vi "InitIntensityGraph.vi"(8 "error in (no error)":errorcluster, 11 "IntensityGraph in":refnum<vi>) -> (0 "error out":errorcluster, 3 "IntensityGraph out":refnum<vi>)   [LabVIEW 2023]
doc: "This VI setups the intensity map and fills it with generated test data for the purpose of this demo."
panel:
  out "appended array":dbl[][](array[numeric])
  in  "Number Y":i32
  in  "StartY":dbl=-0.5
  in  "NumberX":i32
  in  "StartX":dbl=-0.5
  in  "r":dbl
  in  "Y center":dbl
  in  "X center":dbl
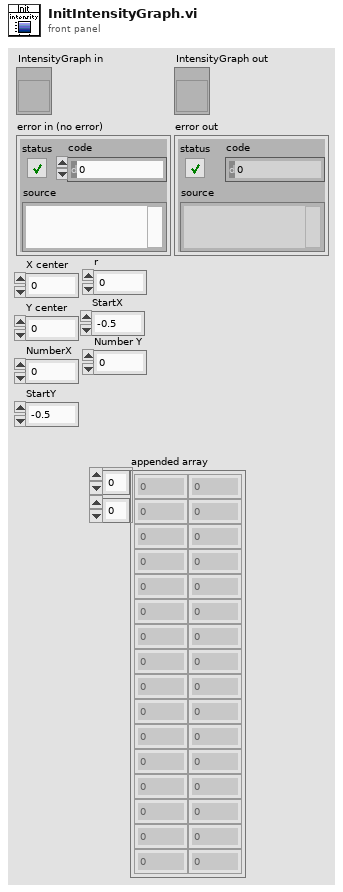
[diagram p1: front panel]
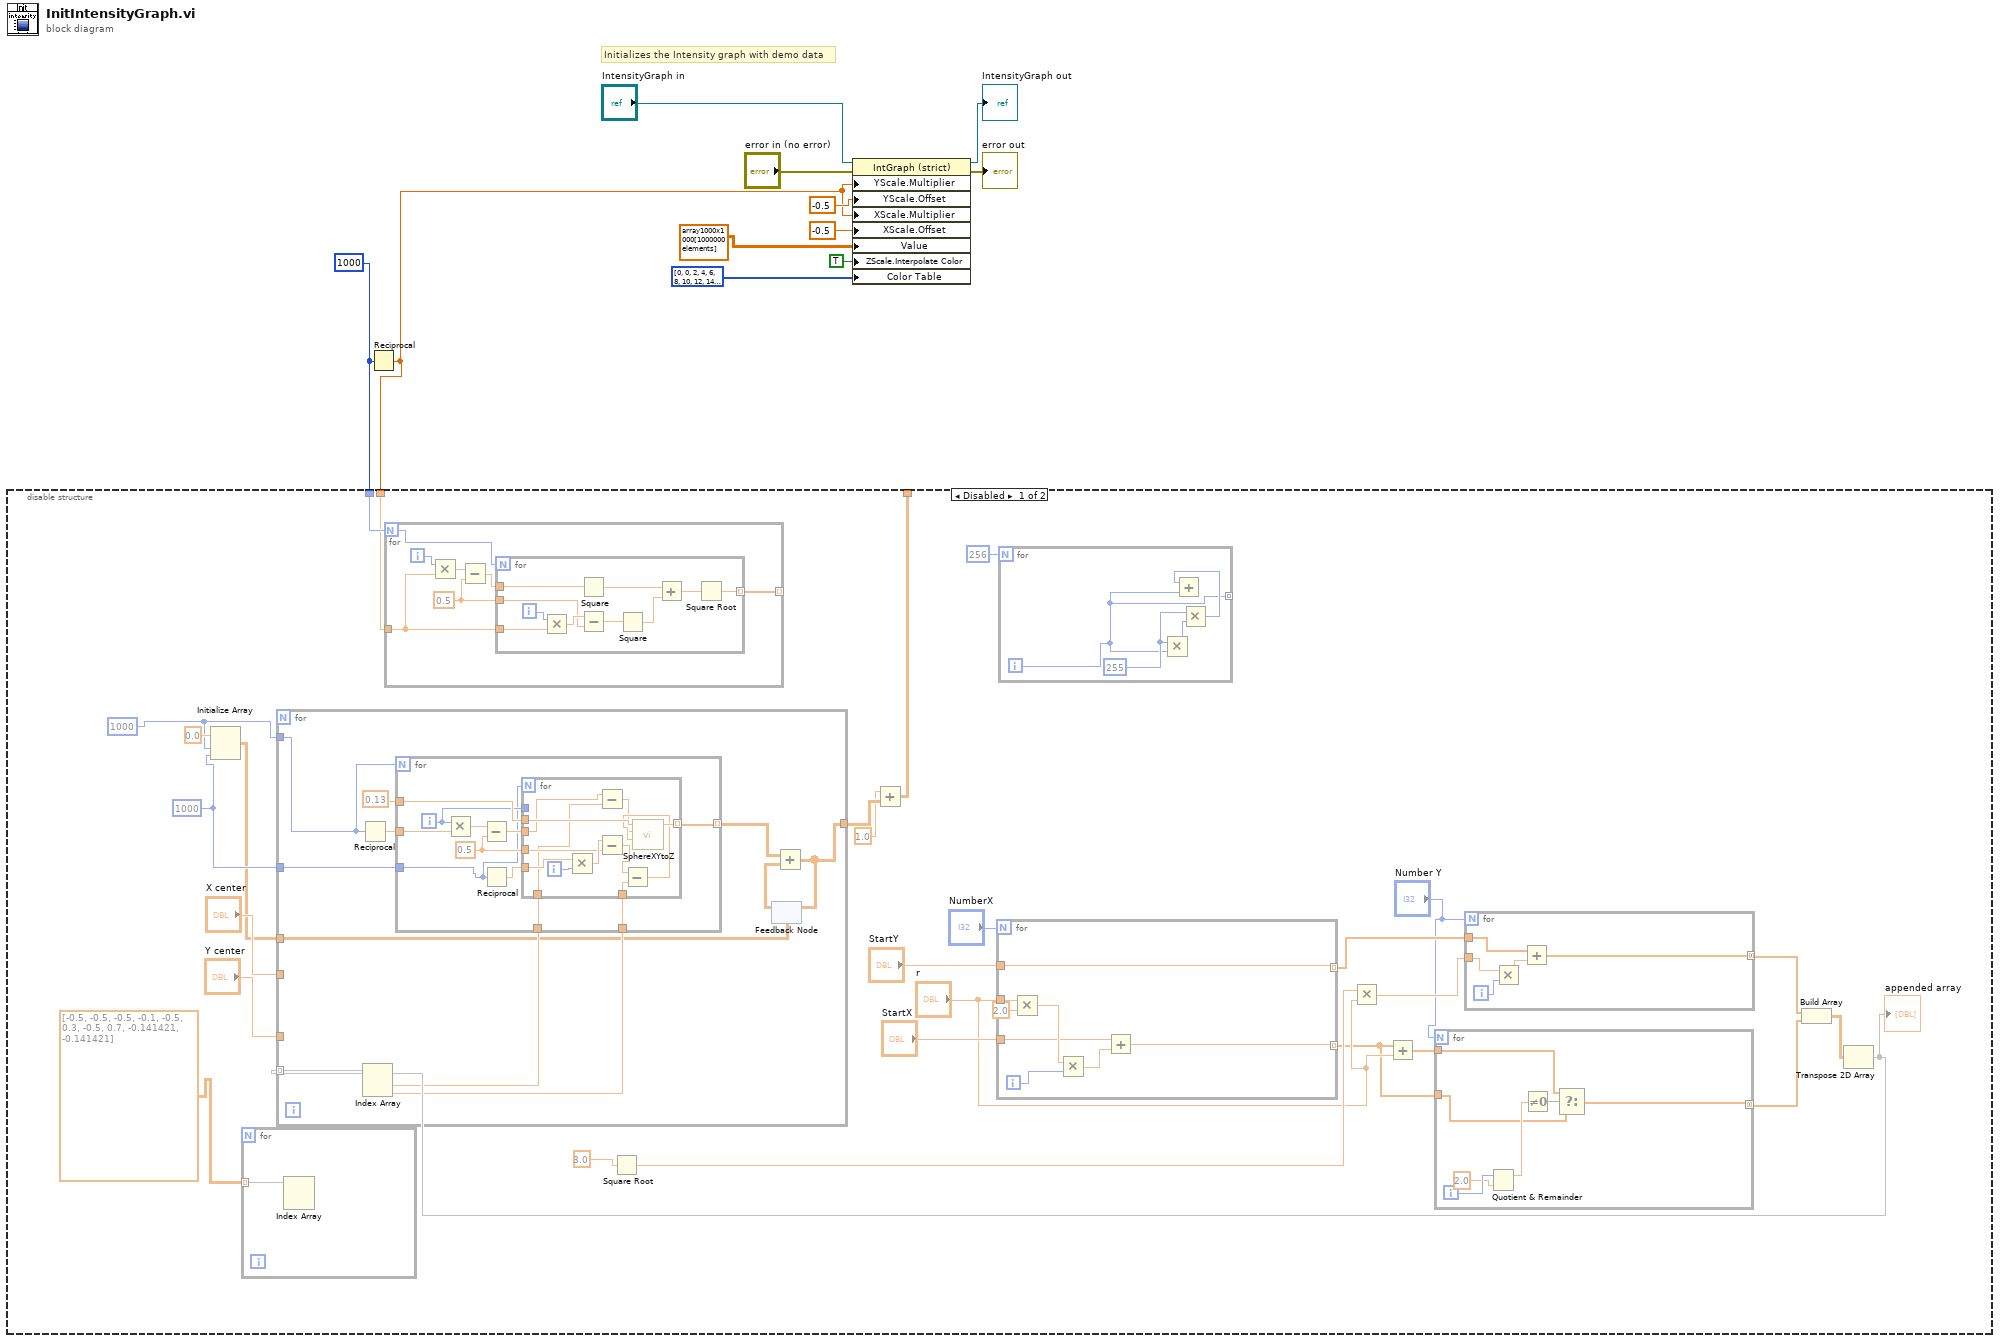
[diagram p0: block diagram]
diagram:
  w3 = 1000
  # "Initializes the Intensity graph with demo data"
  n1 = Reciprocal(x=w3) -> (1/x=w2:dbl)
  n2 = disable-structure shown="Disabled" {
    disable-tunnel: [w38 _] -> _
    disable-tunnel: w3 -> [w14 _]
    disable-tunnel: w2 -> [w13 _]
    frame Disabled {
      w15 = 1000
      w34 = 1000
      n3 = Initialize Array(0.0 ("element"), w15, w34) -> (w32:dbl[][])
      n4 = for {
        tunnel: dbl[][] [[-0.5, -0.5], [-0.5, -0.1], [-0.5, 0.3], [-0.5, 0.7], [-0.141421, -0.141421]] -> [w81] mode=indexing
        n5 = Index Array(array=w81) -> ()  [unwired: 2 in, 2 out]
      }
      n6 = for {
        N: w14 -> [w44]
        tunnel: w13 -> [w49]
        tunnel: [w45] -> _ mode=indexing
        i -> [w50]
        w47 = 0.5 ("y")
        n7 = Multiply(x=w50, y=w49) -> (x*y=w48:dbl)
        n8 = Subtract(x=w48, y=w47) -> (x-y=w46:dbl)
        n9 = for {
          N: w44 -> [_]
          tunnel: w49 -> [w59]
          tunnel: w47 -> [w57]
          tunnel: w46 -> [w55]
          tunnel: [w51] -> w45 mode=indexing
          i -> [w60]
          n10 = Multiply(x=w60, y=w59) -> (x*y=w58:dbl)
          n11 = Square(x=w55) -> (x^2=w53:dbl)
          n12 = Subtract(x=w58, y=w57) -> (x-y=w56:dbl)
          n13 = Square(x=w56) -> (x^2=w54:dbl)
          n14 = Add(x=w53, y=w54) -> (x+y=w52:dbl)
          n15 = Square Root(x=w52) -> (sqrt(x)=w51:dbl)
        }
      }
      n16 = Square Root(x=3.0) -> (sqrt(x)=w26:dbl)
      n17 = for {
        N: "NumberX" -> [_]
        tunnel: "r" -> [w79]
        tunnel: "StartX" -> [w75]
        tunnel: [w74] -> w20 mode=indexing
        tunnel: [w73] -> w24 mode=indexing
        tunnel: "StartY" -> [w73]
        i -> [w80]
        n18 = Multiply(x=w79, y=2.0) -> (x*y=w77:dbl)
        n19 = Multiply(x=w77, y=w80) -> (x*y=w76:dbl)
        n20 = Add(x=w75, y=w76) -> (x+y=w74:dbl)
      }
      n21 = for {
        N: 256 -> [_]
        tunnel: [w40] -> _ mode=indexing
        i -> [w40]
        w43 = 255 ("x")
        n22 = Multiply(x=w43, y=w40) -> (x*y=w42:i32)
        n23 = Multiply(x=w43, y=w42) -> (x*y=w41:i32)
        n24 = Add(x=w41, y=w40) -> ()  [unwired: 1 out]
      }
      n25 = Multiply(x=w26, y="r") -> (x*y=w23:dbl)
      n26 = Add(x=w20, y="r") -> (x+y=w21:dbl[])
      n27 = for {
        N: "Number Y" -> [_]
        tunnel: w21 -> [w68]
        tunnel: w20 -> [w67]
        tunnel: [w66] -> w18 mode=concatenating
        i -> [w72]
        n28 = Quotient & Remainder(x=w72, y=2.0) -> (x-y*floor(x/y)=w69:dbl)  [unwired: 1 out]
        n29 = Not Equal To 0?(x=w69) -> (x != 0?=w70:bool)
        n30 = Select(t=w68, s=w70, f=w67) -> (s? t:f=w66:dbl[])
      }
      n31 = for {
        N: "Number Y" -> [_]
        tunnel: w23 -> [w62]
        tunnel: w24 -> [w65]
        tunnel: [w61] -> w19 mode=concatenating
        i -> [w64]
        n32 = Multiply(x=w62, y=w64) -> (x*y=w63:dbl)
        n33 = Add(x=w65, y=w63) -> (x+y=w61:dbl[])
      }
      n34 = Build Array(w19, w18) -> (w17:dbl[][])
      n35 = Transpose 2D Array(2D array=w17) -> (transposed array=w16:dbl[][])
      "appended array" <- w16
      n36 = for {
        tunnel: [w82] -> w39
        tunnel: "X center" -> [_]
        tunnel: "Y center" -> [_]
        tunnel: w16 -> [w90] mode=indexing
        tunnel: w15 -> [w85]
        tunnel: w34 -> [w86]
        tunnel: w32 -> [w84]
        n37 = Reciprocal(x=w85) -> (1/x=w91:dbl)
        n38 = Index Array(array=w90) -> (element #1=w89:dbl, element #2=w88:dbl)  [unwired: 2 in]
        n39 = for {
          N: w85 -> [_]
          tunnel: 0.13 -> [w103]
          tunnel: w91 -> [w101]
          tunnel: [w96] -> w87 mode=indexing
          tunnel: w89 -> [w95]
          tunnel: w88 -> [w94]
          tunnel: w86 -> [w93]
          i -> [w102]
          w97 = 0.5 ("y")
          n40 = Multiply(x=w102, y=w101) -> (x*y=w99:dbl)
          n41 = Subtract(x=w99, y=w97) -> (x-y=w98:dbl)
          n42 = Reciprocal(x=w93) -> (1/x=w100:dbl)
          n43 = for {
            N: w93 -> [_]
            tunnel: w103 -> [w114]
            tunnel: w102 -> [_]
            tunnel: w98 -> [w109]
            tunnel: [w113] -> w96 mode=indexing
            tunnel: w100 -> [w112]
            tunnel: w97 -> [w110]
            tunnel: w95 -> [w105]
            tunnel: w94 -> [w104]
            i -> [w115]
            n44 = Multiply(x=w112, y=w115) -> (x*y=w111:dbl)
            n45 = Subtract(x=w109, y=w105) -> (x-y=w106:dbl)
            n46 = Subtract(x=w111, y=w110) -> (x-y=w108:dbl)
            n47 = Subtract(x=w108, y=w104) -> (x-y=w107:dbl)
            n48 = call "SphereXYtoZ.vi"("distance from center y"=w107, "Distance from center x"=w106, "Radius"=w114) -> ("distance from center Z"=w113:dbl)  [unwired: 8 in]
          }
        }
        n49 = feedback #1(w84) -> (w83:dbl[][])
        n50 = Add(x=w87, y=w83) -> (x+y=w82:dbl[][])
        n51 = feedback-in #1(w82) -> ()
      }
      n52 = Add(x=1.0, y=w39) -> (x+y=w38:dbl[][])
    }
    frame Enabled {
    }
  }
  n53 = property on="Property Node" class="IntGraph (strict)"(reference="IntensityGraph in", error in="error in (no error)", "YScale.Multiplier"=w2, "YScale.Offset"=-0.5 ("Y Scale.Offset and Multiplier:Offset"), "XScale.Multiplier"=w2, "XScale.Offset"=-0.5 ("X Scale.Offset and Multiplier:Offset"), "Value"=dbl[][] array1000x1000[1000000 elements] ("Intensity Graph"), "ZScale.Interpolate Color"=TRUE ("Z Scale.Interpolate Color"), "Color Table"=u32[] [0, 0, 2, 4, 6, 8, 10, 12, 14, 16, 18, 20, 22, 24, 26, 28, 30, 32, 34, 36, 38, 40, 42, 44, 46, 48, 50, 52, 54, 56, 58, 60, 62, 64, 66, 68, 70, 72, 74, 76, 78, 80, 82, 84, 86, 88, 90, 92, 94, 96, 98, 100, 102, 104, 106, 108, 110, 112, 114, 116, 118, 120, 122, 124, 126, 128, 130, 132, 134, 136, 138, 140, 142, 144, 146, 148, 150, 152, 154, 156, 158, 160, 162, 164, 166, 168, 170, 172, 174, 176, 178, 180, 182, 184, 186, 188, 190, 192, 194, 196, 198, 200, 202, 204, 206, 208, 210, 212, 214, 216, 218, 220, 222, 224, 226, 228, 230, 232, 234, 236, 238, 240, 242, 244, 246, 248, 250, 252, 255, 131839, 263423, 395007, 526591, 658175, 789759, 921343, 1052927, 1184511, 1316095, 1447679, 1579263, 1710847, 1842431, 1974015, 2105599, 2237183, 2368767, 2500351, 2631935, 2763519, 2895103, 3026687, 3158271, 3289855, 3421439, 3553023, 3684607, 3816191, 3947775, 4079359, 4210943, 4342527, 4474111, 4605695, 4737279, 4868863, 5000447, 5132031, 5263615, 5395199, 5526783, 5658367, 5789951, 5921535, 6053119, 6184703, 6316287, 6447871, 6579455, 6711039, 6842623, 6974207, 7105791, 7237375, 7368959, 7500543, 7632127, 7763711, 7895295, 8026879, 8158463, 8290047, 8421631, 8553215, 8684799, 8816383, 8947967, 9079551, 9211135, 9342719, 9474303, 9605887, 9737471, 9869055, 10000639, 10132223, 10263807, 10395391, 10526975, 10658559, 10790143, 10921727, 11053311, 11184895, 11316479, 11448063, 11579647, 11711231, 11842815, 11974399, 12105983, 12237567, 12369151, 12500735, 12632319, 12763903, 12895487, 13027071, 13158655, 13290239, 13421823, 13553407, 13684991, 13816575, 13948159, 14079743, 14211327, 14342911, 14474495, 14606079, 14737663, 14869247, 15000831, 15132415, 15263999, 15395583, 15527167, 15658751, 15790335, 15921919, 16053503, 16185087, 16316671, 16448255, 16579839, 16777215]) -> (reference out=→"IntensityGraph out":refnum<vi>, error out=→"error out":errorcluster)
